vi "SS Get Device.vi"(8 "error in (no error)":errorcluster, 11 "Device Type":string) -> (0 "error out":errorcluster, 3 "Device Name":string)   [LabVIEW 2021]
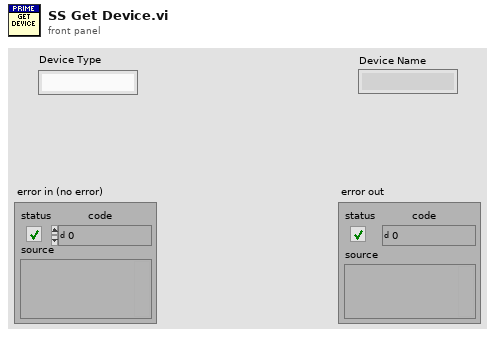
[diagram p1: front panel]
types:
  T1 = typedef "CC cluster Hardware Config.ctl" = cluster{"Installed Hardware":T2[]}
  T2 = typedef "CC cluster Device Index.ctl" = cluster{"Device Type Name":string, "Curr Device Name":string, "All Instances":string[]}
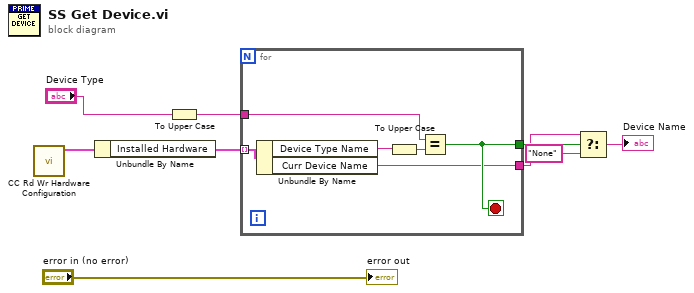
[diagram p0: block diagram]
diagram:
  n1 = call "CC Rd Wr Hardware Configuration.vi"() -> ("Hardware Config out"=w8:T1)  [unwired: 9 in, 2 out]
  n2 = Unbundle By Name(w8) -> ("Installed Hardware"=w7:T2[])
  n3 = To Upper Case(1:"Device Type") -> (0:w5:string)
  n4 = for {
    tunnel: w7 -> [w15] mode=indexing
    tunnel: w5 -> [w12]
    tunnel: [w11] -> w4
    tunnel: [w10] -> w3
    stop <- w11 stop-if-true
    n5 = Unbundle By Name(w15) -> ("Device Type Name"=w14:string, "Curr Device Name"=w10:string)
    n6 = To Upper Case(1:w14) -> (0:w13:string)
    n7 = Equal?(x=w12, y=w13) -> (x = y?=w11:bool)
  }
  n8 = Select(t=w3, s=w4, f="None") -> (s? t:f=→"Device Name":string)
  "error out" <- "error in (no error)"
